vi "Func-교정용 ADC 데이터 수집.vi"(2 "수신 실패(T)":refnum<vi>, 3 "ADC 채널(0~3)":u8, 4 "전송 문자열":string, 5 "Port-act 1":refnum<visa-resource-name>) -> (1 "mean":dbl)   [LabVIEW 2015]
uses:
  <vilib>/Analysis/baseanly.llb/Mean (DBL).vi
  <vilib>/Analysis/NI_AALBase.lvlib
panel:
  out "수신 문자열":string
  out "Loop cnt":i32
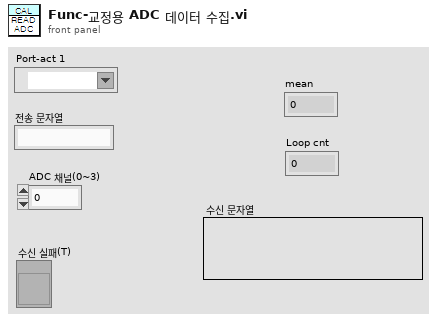
[diagram p1: front panel]
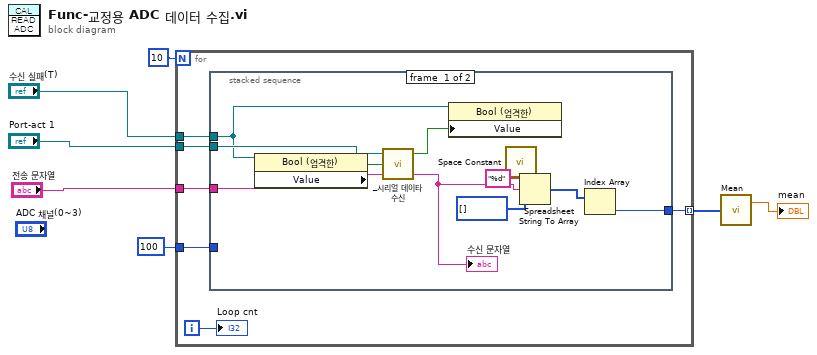
[diagram p0: block diagram]
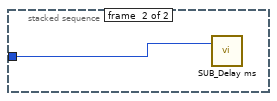
[diagram p2: hidden frame]
diagram:
  n1 = for {
    N: 10 -> [_]
    tunnel: [w13] -> w6 mode=indexing
    tunnel: "Port-act 1" -> [w12]
    tunnel: "전송 문자열" -> [w11]
    tunnel: u32 100 ("ms 배수") -> [w10]
    tunnel: "수신 실패(T)" -> [w9]
    i -> [w8]
    n2 = stacked-sequence {
      tunnel: [w18 _] -> w13
      tunnel: w12 -> [w17 _]
      tunnel: w11 -> [w16 _]
      tunnel: w10 -> [_ w25]
      tunnel: w9 -> [w14 _]
      frame #0 {
        n3 = property class="Bool (엄격한)"(reference=w14) -> ("Value"=w15:bool)  [unwired: 1 in, 2 out]
        n4 = call "_시리얼 데이타 수신.vi"("전송 문자열"=w16, "ErrIn"=w15, "시리얼 포트"=w17) -> ("수신 문자열"=w21:string, "수신 실패(T)"=w23:bool)  [unwired: 1 out]
        "수신 문자열" <- w21
        n5 = property class="Bool (엄격한)"(reference=w14, "Value"=w23) -> ()  [unwired: 1 in, 2 out]
        n6 = call <vilib>:"Space Constant.vi"() -> ("String"=w19:string)
        n7 = Spreadsheet String To Array(delimiter (Tab)=w19, format string="%d" ("포맷 문자열"), spreadsheet string=w21, array type (2D Dbl)=u32[] [] ("배열 타입(2D Dbl)")) -> (array=w24:u32[])
        n8 = Index Array(array=w24) -> (element=w18:u32)  [unwired: 1 in]
      }
      frame #1 {
        n9 = call "SUB_Delay ms.vi"("delay(ms)"=w25) -> ()  [unwired: 3 in]
      }
    }
    "Loop cnt" <- w8
  }
  n10 = call-poly <vilib>:"Mean.vi"("X"=w6) -> ("mean"=→"mean":dbl)  [unwired: 1 out]
